vi "Wind_Turbine.vi"() -> (5 "Plug in titles":string[](array[string]), 7 "Plug in values":string[](array[string]))   [LabVIEW 2010]
uses:
  Globals/Meas_global.vi
  Globals/Plug_in_data_global.vi
  Globals/LDA_meas_global_1.vi
  <vilib>/Analysis/NI_AALBase.lvlib
panel:
  in  "Change Dem Voltages?":bool
  out "All WTs":dbl[][](array[numeric]) format="%#.2g"
  out "WT trace index":i32[](array[numeric])
  in  "precision":string
  in  "Add Phase data to results file":bool
  in  "Separation Character":string="\t"
  in  "Output Directory":path
  in  "Save Phase averaged Profiles":bool
  out "LDA Chs":i32[](array[numeric])
  out "WT Stalled?":bool
  out "Pulse No":i32
  out "Last index":i32
  out "subarray":bool[](array[boolean])
  out "Index":i32[](array[numeric])
  out "Pulses per Rev":i32
  out "Av samples per pulse":i32
  out "Threshold":dbl
  in  "Channel to Phase lock":i32[](listbox)
  out "Last Block No of Revs":i32
  out "Hub RPM":dbl
  out "Generator trace":cluster{dbl, dbl, dbl[]}(graph)
  out "Hot wire trace":cluster{dbl, dbl, dbl[][]}(graph)
  out "Number of Revs":i32
  # "Mean RPM      SD RPM           Max-Min"
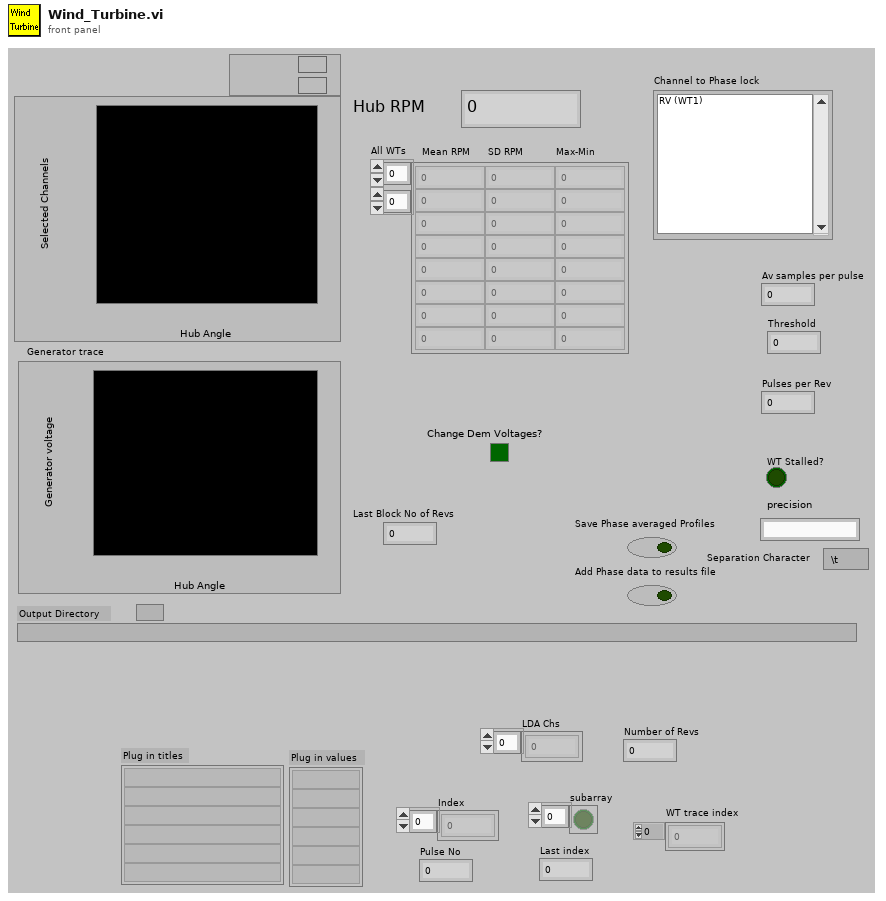
[diagram p1: front panel]
types:
  T1 = typedef "Analysis_info_cluster.ctl" = cluster{"Colour":u32, "Inst type":T2, "Inst name":string, "Symbol":string, "Code name":string, "Extra Info":string, "Inst Array":T3, "Index":i32, "Voltage Index":i32, "Extra Titles":string[], "Extra Values":string[]}
  T2 = typedef "Inst_type.ctl" = enum16{"Propeller anemometer", "Raw voltage", "Pressure Transducer", "Pitot-static tube", "Preston tube", "Hot wire", "Cross wire 1", "Cross wire 2", "Generic Linear", "Generic Polynomial", "Generic BackPoly", "Fast FID", "Thermocouple", "Cold wire", "Pulsed Wire", "LDA Vel", "LDA Tran time", "LDA Arr time"}
  T3 = typedef "Instrument_Array.ctl" = enum16{"PWA", "LDA", "Analogue"}
  T4 = typedef "Post_Process.ctl" = enum16{"Take New Data", "Post Process Raw Data File"}
  T5 = cluster{"[0]":bool, "[1]":bool, "[2]":bool, "[3]":bool}
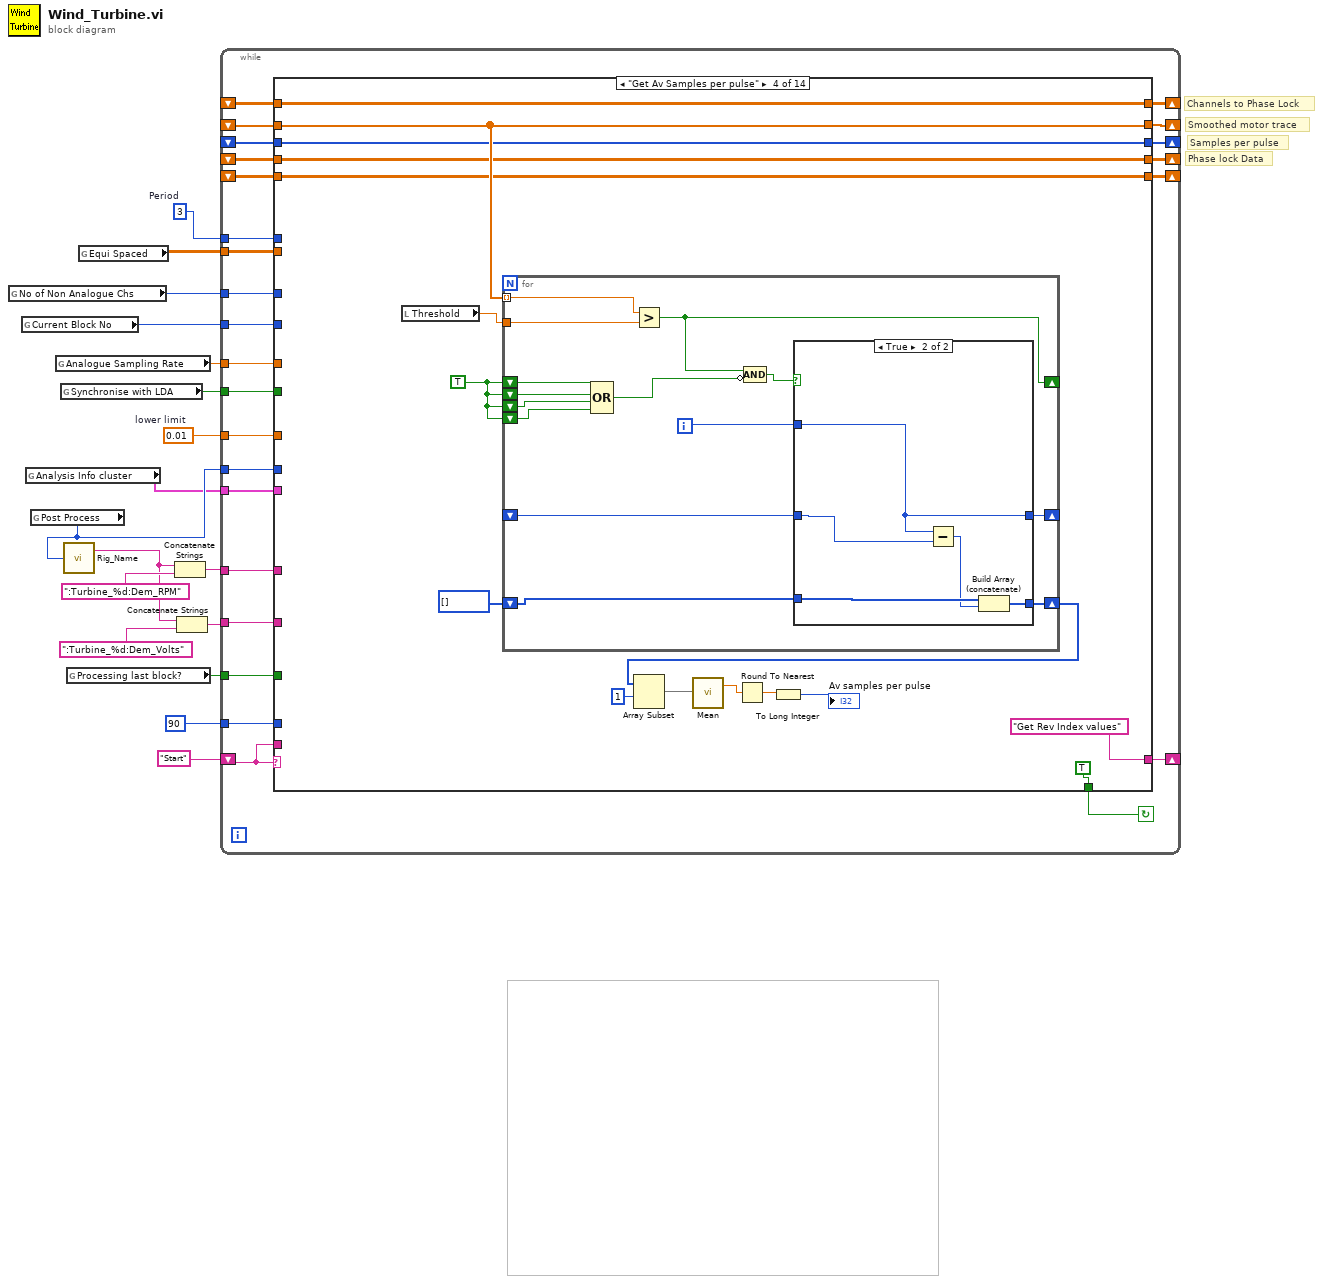
[diagram p0: block diagram]
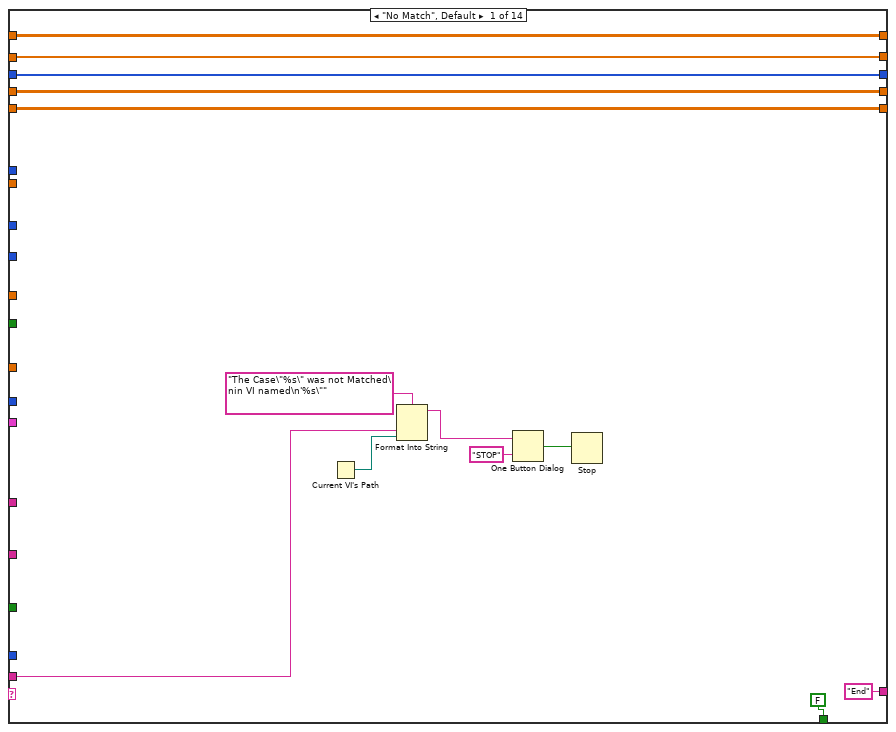
[diagram p2: hidden frame]
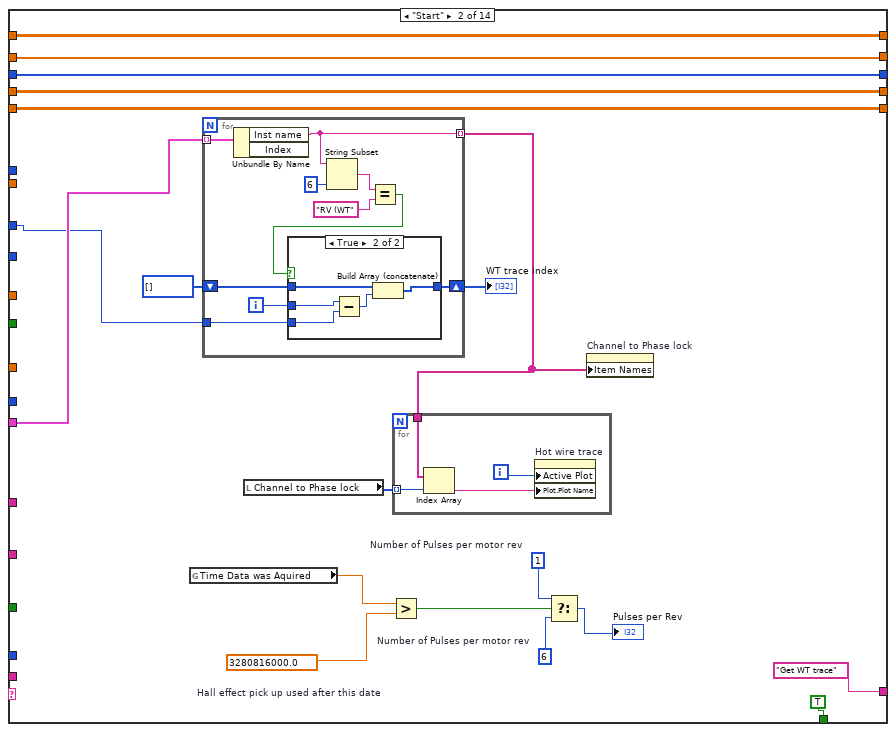
[diagram p3: hidden frame]
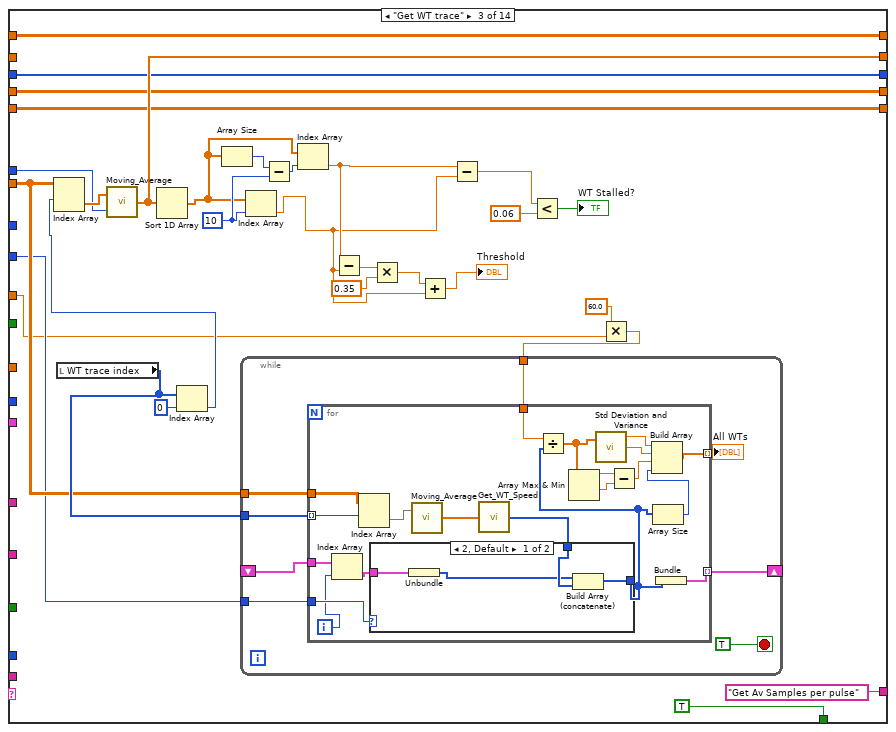
[diagram p5: hidden frame]
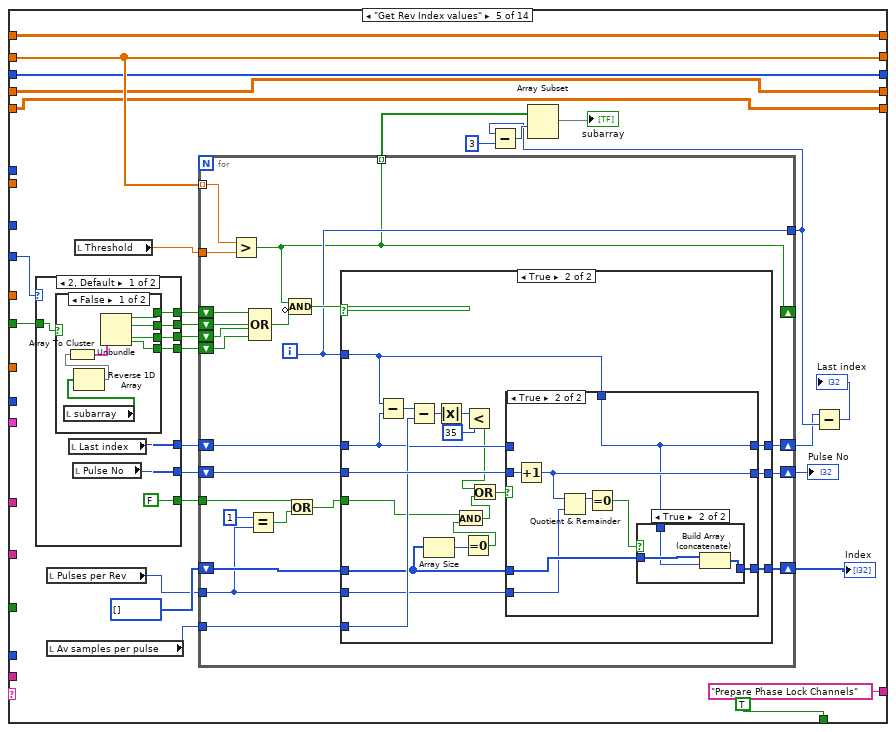
[diagram p8: hidden frame]
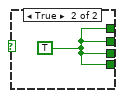
[diagram p9: hidden frame]
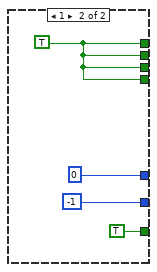
[diagram p10: hidden frame]
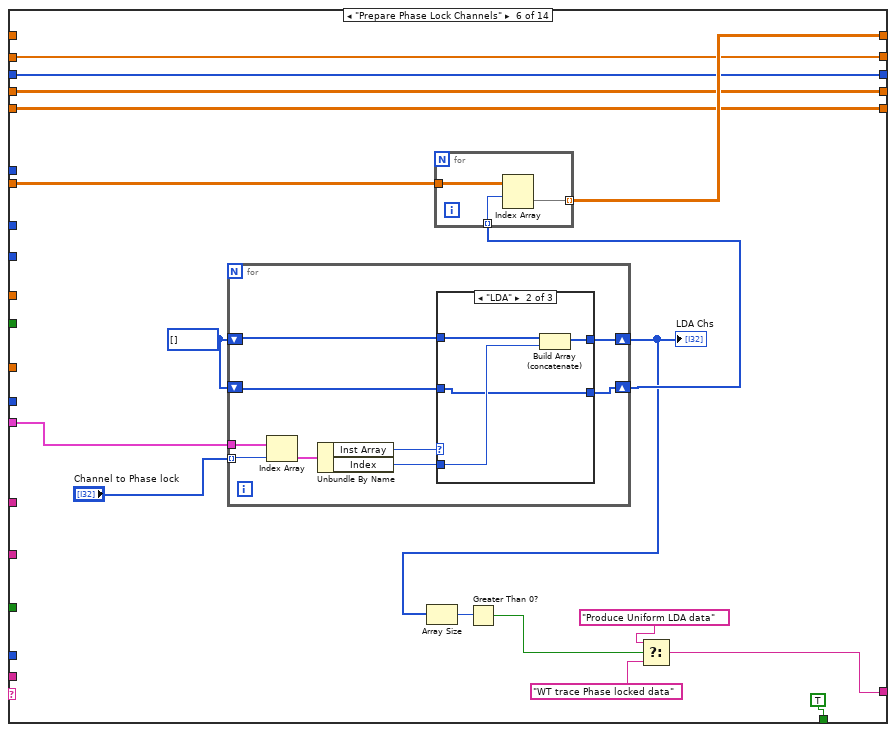
[diagram p14: hidden frame]
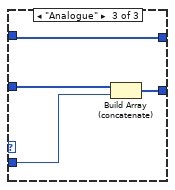
[diagram p16: hidden frame]
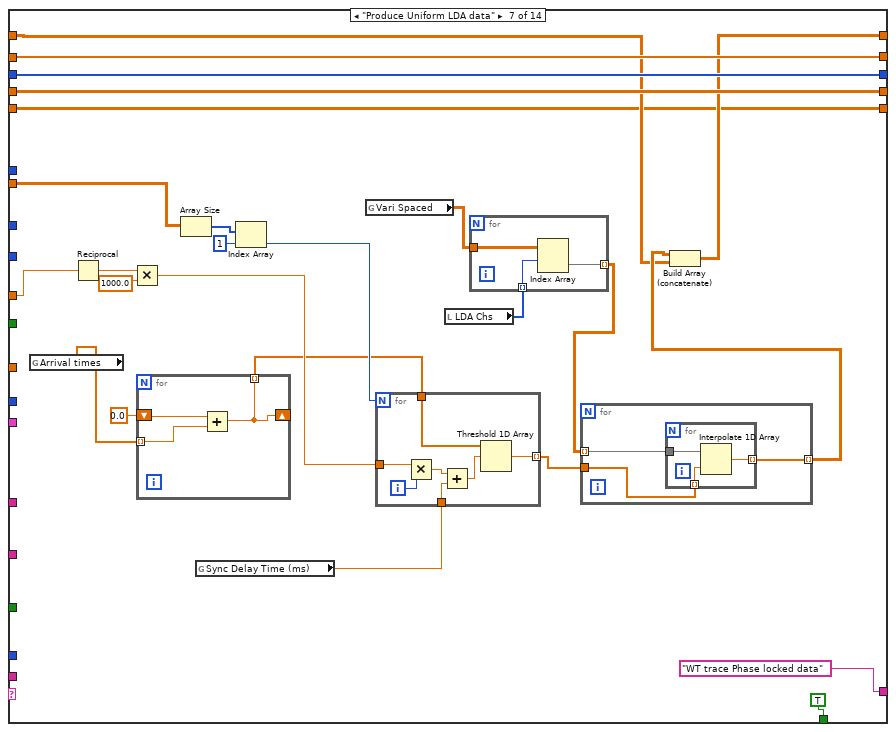
[diagram p17: hidden frame]
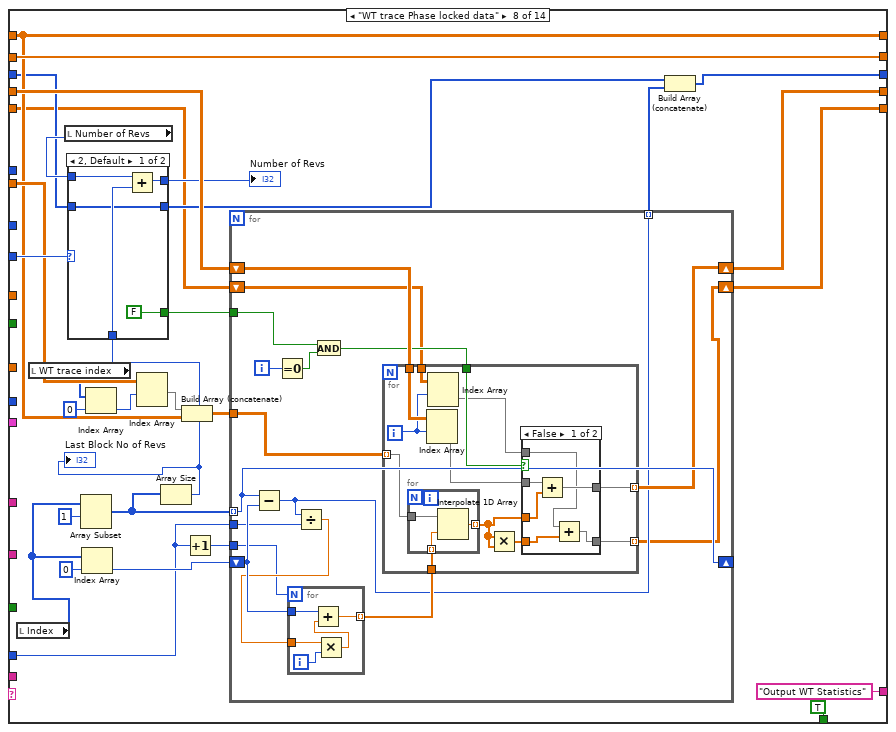
[diagram p18: hidden frame]
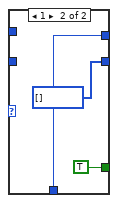
[diagram p19: hidden frame]
diagram:
  w14 = 3  # Period
  w15 = 0.01  # lower limit
  # "Channels to Phase Lock"
  # "Phase lock Data"
  # "Samples per pulse"
  # "Smoothed motor trace"
  n1 = global read "Meas_global.vi" "No of Non Analogue Chs"() -> (w3:i32)
  n2 = global read "Meas_global.vi" "Current Block No"() -> (w17:i32)
  n3 = global read "Meas_global.vi" "Analysis Info cluster"() -> (w6:T1[])
  n4 = global read "Meas_global.vi" "Post Process"() -> (w13:T4)
  n5 = global read "Meas_global.vi" "Analogue Sampling Rate"() -> (w16:dbl)
  n6 = global read "Meas_global.vi" "Synchronise with LDA"() -> (w7:bool)
  n7 = call "Rig_Name.vi"("Post Process"=w13) -> ("Rig Setup before dash"=w9:string)  [unwired: 1 out]
  n8 = global read "Meas_global.vi" "Processing last block?"() -> (w4:bool)
  n9 = global read "Plug_in_data_global.vi" "Equi Spaced"() -> (w2:dbl[][])
  n10 = Concatenate Strings(w9, ":Turbine_%d:Dem_RPM") -> (w8:string)
  n11 = Concatenate Strings(w9, ":Turbine_%d:Dem_Volts") -> (w12:string)
  n12 = while {
    tunnel: w17 -> [w43]
    tunnel: w2 -> [w42]
    shift-right: [w40] -> _
    shift-left: _ -> [w41]
    shift-right: [w39] -> _
    shift-left: _ -> [w38]
    tunnel: w16 -> [w37]
    tunnel: w12 -> [w36]
    tunnel: w8 -> [w35]
    tunnel: w15 -> [w34]
    tunnel: w14 -> [w33]
    tunnel: w13 -> [w32]
    tunnel: w7 -> [w31]
    tunnel: w6 -> [w30]
    shift-right: [w29] -> _
    shift-left: _ -> [w28]
    shift-right: [w27] -> _
    shift-left: "Start" -> [w25]
    tunnel: w4 -> [w24]
    tunnel: w3 -> [w23]
    shift-right: [w22] -> _
    shift-left: _ -> [w21]
    tunnel: 90 -> [w20]
    shift-right: [w18] -> _
    shift-left: _ -> [w19]
    stop <- w26 continue-if-true
    n13 = case shown="\"Get Av Samples per pulse\"" w25 {
      tunnel: w43 -> [_ _ w105 _ w223 _ _ w414 _ _ _ _ _ _]
      tunnel: w42 -> [_ _ w106 _ _ w316 w356 w410 _ _ _ _ _ _]
      tunnel: w41 -> [w48 w64 w112 w161 w200 w312 w365 w409 w485 w529 w570 w597 w671 w685]
      tunnel: [w48 w64 w112 w161 w200 w312 w365 w408 w485 w529 w570 w597 w671 w685] -> w40
      tunnel: [w49 w65 w113 w162 w201 w313 w366 w404 w494 w527 w568 w605 w672 w690] -> w39
      tunnel: w38 -> [w49 w65 w113 w162 w201 w313 w366 w394 w494 w527 w568 w605 w672 w690]
      tunnel: w37 -> [_ _ w103 _ _ _ w359 _ w498 _ _ _ _ w689]
      tunnel: w36 -> [_ _ _ _ _ _ _ _ _ w534 w566 _ _ _]
      tunnel: w35 -> [_ _ _ _ _ _ _ _ _ w533 w541 _ _ _]
      tunnel: w34 -> [_ _ _ _ _ _ _ _ _ _ _ _ _ _]
      tunnel: w33 -> [_ _ w124 _ _ _ _ _ _ _ _ _ _ _]
      tunnel: w32 -> [_ _ _ _ _ _ _ _ _ w532 _ _ _ _]
      tunnel: w31 -> [_ _ _ _ w208 _ _ _ _ _ _ _ _ _]
      tunnel: w30 -> [_ w69 _ _ _ w320 _ _ _ _ _ _ _ _]
      tunnel: [w50 w66 w117 w163 w202 w314 w367 w403 w493 w530 w571 w606 w673 w691] -> w29
      tunnel: w28 -> [w50 w66 _ w163 w202 w314 w367 w403 w493 w530 w571 w606 w673 w691]
      tunnel: ["End" "Get WT trace" "Get Av Samples per pulse" "Get Rev Index values" "Prepare Phase Lock Channels" w308 "WT trace Phase locked data" ("f") "Output WT Statistics" "Get Last Block info" w531 "End" ("f") "Check Folder Name" "Save Phase locked data" "End"] -> w27
      tunnel: [FALSE ("Change Control Voltage?") TRUE ("Processing last block?") TRUE TRUE ("Processing last block?") TRUE ("Change Control Voltage?") TRUE ("Change Control Voltage?") TRUE ("Change Control Voltage?") TRUE ("Change Control Voltage?") TRUE ("Change Control Voltage?") w525 FALSE ("Change Control Voltage?") w602 w663 FALSE ("Change Control Voltage?")] -> w26
      tunnel: w25 -> [w51 _ _ _ _ _ _ _ _ _ _ _ _ _]
      tunnel: w24 -> [_ _ _ _ _ _ _ _ _ w524 _ w600 _ _]
      tunnel: w23 -> [_ w57 _ _ _ _ _ _ _ _ _ _ _ _]
      tunnel: [w45 w63 w111 w160 w197 w315 w345 w398 w486 w528 w569 w604 w670 w688] -> w22
      tunnel: w21 -> [w45 w63 w111 w160 w197 _ w347 w398 w486 w528 w569 w604 w670 w688]
      tunnel: w20 -> [_ _ _ _ _ _ _ w397 w481 _ _ w598 _ w683]
      tunnel: w19 -> [w44 w60 w110 w159 w196 w304 w343 w391 w475 w526 w567 w596 w661 w684]
      tunnel: [w44 w60 w110 w159 w196 w304 w343 w390 w475 w526 w567 w596 w661 w684] -> w18
      frame "No Match", Default {
        n14 = Current VI's Path() -> (path=w52:path)
        n15 = Format Into String(format string="The Case\"%s\" was not Matched\nin VI named\n'%s\"" ("Format String"), w51, w52) -> (resulting string=w55:string)  [unwired: 2 in, 1 out]
        n16 = One Button Dialog(message=w55, button name ("OK")="STOP") -> (true=w53:bool)
        n17 = Stop(stop? (T)=w53) -> ()
      }
      frame "Start" {
        w70 = 6  # Number of Pulses per motor rev
        w71 = 1  # Number of Pulses per motor rev
        w73 = 3280816000.0  # Hall effect pick up used after this date
        n18 = global read "Meas_global.vi" "Time Data was Aquired"() -> (w74:dbl)
        n19 = for {
          tunnel: w69 -> [w89] mode=indexing
          tunnel: [w88] -> w62 mode=indexing
          shift-right: [w82] -> w58
          shift-left: i32[] [] -> [w83]
          tunnel: w57 -> [w80]
          i -> [w81]
          n20 = Unbundle By Name(w89) -> ("Inst name"=w88:string)  [unwired: 1 out]
          n21 = String Subset(string=w88, length (rest)=6 ("length (rest)")) -> (substring=w85:string)  [unwired: 1 out]
          n22 = Equal?(x=w85, y="RV (WT") -> (x = y?=w84:bool)
          n23 = case shown="True" w84 {
            tunnel: w83 -> [w90 w95]
            tunnel: [w90 w94] -> w82
            tunnel: w81 -> [_ w93]
            tunnel: w80 -> [_ w91]
            frame False {
            }
            frame True {
              n24 = Subtract(x=w93, y=w91) -> (x-y=w92:i32)
              n25 = Build Array (concatenate)(w95, w92) -> (w94:i32[])
            }
          }
        }
        "WT trace index" <- w58
        n26 = local read "Channel to Phase lock"() -> (w61:i32[])
        n27 = Greater?(x=w74, y=w73) -> (0:w72:bool)
        n28 = for {
          tunnel: w62 -> [w79]
          tunnel: w61 -> [w78] mode=indexing
          i -> [w77]
          n29 = Index Array(array=w79, index=w78) -> (element=w76:string)
          n30 = property on="Hot wire trace" class="WFGraph (strict)"("Active Plot"=w77, "Plot.Plot Name"=w76) -> ()  [unwired: 2 in, 2 out]
        }
        n31 = Select(t=w71, s=w72, f=w70) -> (s? t:f=→"Pulses per Rev":i32)
        n32 = property on="Channel to Phase lock" class="LstBox (strict)"("Item Names"=w62) -> ()  [unwired: 2 in, 2 out]
      }
      frame "Get WT trace" {
        w122 = 10 ("index")
        n33 = local read "WT trace index"() -> (w107:i32[])
        n34 = Index Array(array=w107, index=0) -> (element=w108:i32)
        n35 = Index Array(array=w106, index (row)=w108) -> (element=w125:dbl[])  [unwired: 1 in]
        n36 = call "Moving_Average.vi"("Period"=w124, "Input Array"=w125) -> ("N+1-Period"=w117:dbl[])
        n37 = Sort 1D Array(array=w117) -> (sorted array=w120:dbl[])
        n38 = Array Size(array=w120) -> (size(s)=w123:i32)
        n39 = Index Array(array=w120, index=w122) -> (element=w97:dbl)
        n40 = Subtract(x=w123, y=w122) -> (x-y=w121:i32)
        n41 = Index Array(array=w120, index=w121) -> (element=w98:dbl)
        n42 = Subtract(x=w98, y=w97) -> (x-y=w101:dbl)
        n43 = Multiply(x=w101, y=0.35) -> (x*y=w99:dbl)
        n44 = Add(x=w99, y=w97) -> (x+y=→"Threshold":dbl)
        n45 = Subtract(x=w98, y=w97) -> (x-y=w118:dbl)
        n46 = Less?(x=w118, y=0.06) -> (x < y?=→"WT Stalled?":bool)
        n47 = Multiply(x=60.0, y=w103) -> (x*y=w102:dbl)
        n48 = while {
          tunnel: w107 -> [w133]
          tunnel: w106 -> [w132]
          tunnel: w105 -> [w131]
          shift-right: [w126] -> _
          shift-left: _ -> [w130]
          tunnel: w102 -> [w129]
          stop <- TRUE stop-if-true
          n49 = for {
            tunnel: w133 -> [w152] mode=indexing
            tunnel: w132 -> [w151]
            tunnel: w131 -> [w149]
            tunnel: w130 -> [w139]
            tunnel: w129 -> [w147]
            tunnel: [w140] -> w127 mode=indexing
            tunnel: [w134] -> w126 mode=indexing
            i -> [w138]
            n50 = Index Array(array=w139, index=w138) -> (element=w137:cluster{"Samples per pulse":i32[]})
            n51 = Index Array(array=w151, index (row)=w152) -> (element=w153:dbl[])  [unwired: 1 in]
            n52 = call "Moving_Average.vi"("Input Array"=w153) -> ("N+1-Period"=w150:dbl[])  [unwired: 1 in]
            n53 = call "Get_WT_Speed.vi"("Opto Trace"=w150) -> ("Samples per pulse"=w148:i32[])
            n54 = case shown="2, Default" w149 {
              tunnel: [w156 w158] -> w135
              tunnel: w148 -> [w157 w158]
              tunnel: w137 -> [w155 _]
              frame 2, Default {
                n55 = Unbundle(w155) -> ("Samples per pulse"=w154:i32[])
                n56 = Build Array (concatenate)(w154, w157) -> (w156:i32[])
              }
              frame 1 {
              }
            }
            n57 = Divide(x=w147, y=w135) -> (x/y=w144:dbl[])
            n58 = Array Max & Min(array=w144) -> (max value=w146:dbl, min value=w145:dbl)  [unwired: 2 out]
            n59 = call <vilib>:"Std Deviation and Variance.vi"("X"=w144) -> ("mean"=w143:dbl, "standard deviation"=w142:dbl)  [unwired: 1 in, 1 out]
            n60 = Subtract(x=w146, y=w145) -> (x-y=w141:dbl)
            n61 = Array Size(array=w135) -> (size(s)=w136:i32)
            n62 = Build Array(w143, w142, w141, w136) -> (w140:dbl[])
            n63 = Bundle("Samples per pulse"=w135) -> (w134:cluster{"Samples per pulse":i32[]})  [unwired: 1 in]
          }
          "All WTs" <- w127
        }
      }
      frame "Get Av Samples per pulse" {
        w172 = TRUE
        n64 = local read "Threshold"() -> (w166:dbl)
        n65 = for {
          shift-right: [w175] -> _
          shift-left: w172 -> [w180]
          shift-right: [w185] -> _
          shift-left: _ -> [w184]
          tunnel: w163 -> [w188] mode=indexing
          tunnel: w166 -> [w187]
          shift-right: [w182] -> w171
          shift-left: i32[] [] -> [w183]
          shift-left: w172 -> [w179]
          shift-left: w172 -> [w178]
          shift-left: w172 -> [w176]
          i -> [w181]
          n66 = Compound Arithmetic op=OR(w180, w179, w178, w176) -> (w177:bool)
          n67 = Greater?(x=w188, y=w187) -> (0:w175:bool)
          n68 = Compound Arithmetic op=AND(w175, invert w177) -> (w186:bool)
          n69 = case shown="True" w186 {
            tunnel: [w190 w193] -> w185
            tunnel: w181 -> [_ w193]
            tunnel: w184 -> [w190 w192]
            tunnel: w183 -> [w189 w195]
            tunnel: [w189 w194] -> w182
            frame False {
            }
            frame True {
              n70 = Subtract(x=w193, y=w192) -> (x-y=w191:i32)
              n71 = Build Array (concatenate)(w195, w191) -> (w194:i32[])
            }
          }
        }
        n72 = Array Subset(array=w171, index=1) -> (w169:i32[])  [unwired: 1 in]
        n73 = call <vilib>:"Mean.vi"("X"=w169) -> ("mean"=w168:dbl)  [unwired: 1 out]
        n74 = Round To Nearest(number=w168) -> (nearest integer value=w167:dbl)
        n75 = To Long Integer(number=w167) -> (32bit integer=→"Av samples per pulse":i32)
      }
      frame "Get Rev Index values" {
        n76 = case shown="2, Default" w223 {
          tunnel: [w225 -1] -> w222
          tunnel: [w226 0] -> w220
          tunnel: [w232 w241] -> w215
          tunnel: [w231 w241] -> w214
          tunnel: [w230 w241] -> w213
          tunnel: [w229 w241] -> w212
          tunnel: [FALSE TRUE] -> w211
          tunnel: w208 -> [w227 _]
          frame 2, Default {
            n77 = case shown="False" w227 {
              tunnel: [w237 w240] -> w232
              tunnel: [w236 w240] -> w231
              tunnel: [w235 w240] -> w230
              tunnel: [w234 w240] -> w229
              frame False {
                n78 = local read "subarray"() -> (w233:bool[])
                n79 = Reverse 1D Array(array=w233) -> (reversed array=w239:bool[])
                n80 = Array To Cluster(array=w239) -> (cluster=w238:T5)
                n81 = Unbundle(w238) -> ("[0]"=w237:bool, "[1]"=w236:bool, "[2]"=w235:bool, "[3]"=w234:bool)
              }
              frame True {
                w240 = TRUE ("[0]")
              }
            }
            n82 = local read "Last index"() -> (w226:i32)
            n83 = local read "Pulse No"() -> (w225:i32)
          }
          frame 1 {
            w241 = TRUE
          }
        }
        n84 = local read "Pulses per Rev"() -> (w205:i32)
        n85 = local read "Av samples per pulse"() -> (w206:i32)
        n86 = local read "Threshold"() -> (w207:dbl)
        n87 = for {
          shift-right: [w252] -> _
          shift-left: w215 -> [w256]
          shift-right: [w263] -> w209
          shift-left: w220 -> [w260]
          tunnel: w202 -> [w266] mode=indexing
          tunnel: w207 -> [w265]
          shift-right: [w261] -> w203
          shift-left: w222 -> [w262]
          shift-right: [w258] -> w204
          shift-left: i32[] [] -> [w259]
          tunnel: [w257] -> w210
          shift-left: w214 -> [w255]
          shift-left: w213 -> [w254]
          tunnel: [w252] -> w217 mode=indexing
          shift-left: w212 -> [w251]
          tunnel: w206 -> [w250]
          tunnel: w211 -> [w246]
          tunnel: w205 -> [w249]
          i -> [w257]
          n88 = Greater?(x=w266, y=w265) -> (0:w252:bool)
          n89 = Equal?(x=1, y=w249) -> (x = y?=w247:bool)
          n90 = Compound Arithmetic op=OR(w256, w255, w254, w251) -> (w253:bool)
          n91 = Or(x=w246, y=w247) -> (x .or. y?=w245:bool)
          n92 = Compound Arithmetic op=AND(w252, invert w253) -> (w264:bool)
          n93 = case shown="True" w264 {
            tunnel: [w269 w279] -> w263
            tunnel: w257 -> [_ w285]
            tunnel: w262 -> [w268 w288]
            tunnel: [w268 w287] -> w261
            tunnel: w260 -> [w269 w278]
            tunnel: w259 -> [w267 w277]
            tunnel: [w267 w286] -> w258
            tunnel: w250 -> [_ w283]
            tunnel: w245 -> [_ w272]
            tunnel: w249 -> [_ w271]
            frame False {
            }
            frame True {
              n94 = Subtract(x=w285, y=w278) -> (x-y=w284:i32)
              n95 = Subtract(x=w284, y=w283) -> (x-y=w282:i32)
              n96 = Array Size(array=w277) -> (size(s)=w275:i32)
              n97 = Absolute Value(x=w282) -> (abs(x)=w281:i32)
              n98 = Equal To 0?(x=w275) -> (x = 0?=w274:bool)
              n99 = And(x=w272, y=w274) -> (x .and. y?=w273:bool)
              n100 = Less?(x=w281, y=35) -> (x < y?=w270:bool)
              n101 = Or(x=w270, y=w273) -> (x .or. y?=w276:bool)
              n102 = case shown="True" w276 {
                tunnel: w288 -> [w291 w299]
                tunnel: [w291 w298] -> w287
                tunnel: w277 -> [w290 w295]
                tunnel: [w290 w294] -> w286
                tunnel: w285 -> [_ w293]
                tunnel: [w289 w293] -> w279
                tunnel: w278 -> [w289 _]
                tunnel: w271 -> [_ w292]
                frame False {
                }
                frame True {
                  n103 = Increment(x=w299) -> (x+1=w298:i32)
                  n104 = Quotient & Remainder(x=w298, y=w292) -> (x-y*floor(x/y)=w297:i32)  [unwired: 1 out]
                  n105 = Equal To 0?(x=w297) -> (x = 0?=w296:bool)
                  n106 = case shown="True" w296 {
                    tunnel: w295 -> [w300 w303]
                    tunnel: w293 -> [_ w302]
                    tunnel: [w300 w301] -> w294
                    frame False {
                    }
                    frame True {
                      n107 = Build Array (concatenate)(w303, w302) -> (w301:i32[])
                    }
                  }
                }
              }
            }
          }
        }
        "Index" <- w204
        "Pulse No" <- w203
        n108 = Subtract(x=w210, y=3) -> (x-y=w218:i32)
        n109 = Array Subset(array=w217, index=w218) -> (→"subarray":bool[])  [unwired: 1 in]
        n110 = Subtract(x=w209, y=w210) -> (x-y=→"Last index":i32)
      }
      frame "Prepare Phase Lock Channels" {
        w318 = i32[] []
        n111 = for {
          tunnel: "Channel to Phase lock" -> [w332] mode=indexing
          tunnel: w320 -> [w331]
          shift-right: [w324] -> w317
          shift-left: w318 -> [w325]
          shift-right: [w326] -> w310
          shift-left: w318 -> [w327]
          n112 = Index Array(array=w331, index=w332) -> (element=w330:T1)
          n113 = Unbundle By Name(w330) -> ("Inst Array"=w329:T3, "Index"=w328:i32)
          n114 = case shown="\"LDA\"" w329 {
            tunnel: w328 -> [_ w338 w342]
            tunnel: w327 -> [w334 w337 w339]
            tunnel: [w334 w336 w339] -> w326
            tunnel: w325 -> [w333 w335 w341]
            tunnel: [w333 w335 w340] -> w324
            frame "PWA" {
            }
            frame "LDA" {
              n115 = Build Array (concatenate)(w337, w338) -> (w336:i32[])
            }
            frame "Analogue" {
              n116 = Build Array (concatenate)(w341, w342) -> (w340:i32[])
            }
          }
        }
        "LDA Chs" <- w310
        n117 = Array Size(array=w310) -> (size(s)=w311:i32)
        n118 = for {
          tunnel: w317 -> [w323] mode=indexing
          tunnel: w316 -> [w322]
          tunnel: [w321] -> w315 mode=indexing
          n119 = Index Array(array=w322, index (row)=w323) -> (element=w321:dbl[])  [unwired: 1 in]
        }
        n120 = Greater Than 0?(x=w311) -> (x > 0?=w309:bool)
        n121 = Select(t="Produce Uniform LDA data", s=w309, f="WT trace Phase locked data") -> (s? t:f=w308:string)
      }
      frame "Produce Uniform LDA data" {
        n122 = global read "LDA_meas_global_1.vi" "Arrival times"() -> (w361:dbl[])
        n123 = Reciprocal(x=w359) -> (1/x=w360:dbl)
        n124 = Multiply(x=w360, y=1000.0) -> (x*y=w357:dbl)
        n125 = for {
          shift-right: [w381] -> _
          shift-left: 0.0 -> [w383]
          tunnel: w361 -> [w382] mode=indexing
          tunnel: [w381] -> w346 mode=indexing
          n126 = Add(x=w383, y=w382) -> (x+y=w381:dbl)
        }
        n127 = Array Size(array=w356) -> (size(s)=w355:i32[])
        n128 = global read "LDA_meas_global_1.vi" "Sync Delay Time (ms)"() -> (w344:dbl)
        n129 = Index Array(array=w355, index=1) -> (element=w353:i32)
        n130 = global read "Plug_in_data_global.vi" "Vari Spaced"() -> (w350:dbl[][])
        n131 = for {
          N: w353 -> [_]
          tunnel: w357 -> [w379]
          tunnel: w346 -> [w378]
          tunnel: [w377] -> w352 mode=indexing
          tunnel: w344 -> [w374]
          i -> [w380]
          n132 = Multiply(x=w379, y=w380) -> (x*y=w376:dbl)
          n133 = Add(x=w376, y=w374) -> (x+y=w375:dbl)
          n134 = Threshold 1D Array(2:w375, 3:w378) -> (0:w377:dbl)  [unwired: 1 out]
        }
        n135 = local read "LDA Chs"() -> (w351:i32[])
        n136 = for {
          tunnel: w351 -> [w386] mode=indexing
          tunnel: w350 -> [w385]
          tunnel: [w384] -> w349 mode=indexing
          n137 = Index Array(array=w385, index (row)=w386) -> (element=w384:dbl[])  [unwired: 1 in]
        }
        n138 = for {
          tunnel: [w370] -> w348 mode=indexing
          tunnel: w349 -> [w369] mode=indexing
          tunnel: w352 -> [w368]
          n139 = for {
            tunnel: [w373] -> w370 mode=indexing
            tunnel: w369 -> [w372]
            tunnel: w368 -> [w371] mode=indexing
            n140 = Interpolate 1D Array(1:w371, 2:w372) -> (0:w373:dbl)
          }
        }
        n141 = Build Array (concatenate)(w348, w347) -> (w345:dbl[][])
      }
      frame "WT trace Phase locked data" {
        n142 = local read "Index"() -> (w406:i32[])
        n143 = local read "WT trace index"() -> (w389:i32[])
        n144 = local read "Number of Revs"() -> (w407:i32)
        n145 = Array Subset(array=w406, index=1) -> (w413:i32[])  [unwired: 1 in]
        n146 = Index Array(array=w406, index=0) -> (element=w412:i32)
        n147 = Index Array(array=w389, index=0) -> (element=w387:i32)
        n148 = Index Array(array=w410, index (row)=w387) -> (element=w400:dbl[])  [unwired: 1 in]
        n149 = Array Size(array=w413) -> (size(s)=w392:i32)
        "Last Block No of Revs" <- w392
        n150 = case shown="2, Default" w414 {
          tunnel: [w419 w424] -> w405
          tunnel: w392 -> [w420 w424]
          tunnel: w407 -> [w421 _]
          tunnel: [FALSE TRUE] -> w411
          tunnel: [w417 i32[] []] -> w395
          tunnel: w394 -> [w417 _]
          frame 2, Default {
            n151 = Add(x=w421, y=w420) -> (x+y=w419:i32)
          }
          frame 1 {
          }
        }
        "Number of Revs" <- w405
        n152 = Build Array (concatenate)(w400, w398) -> (w399:dbl[][])
        n153 = Increment(x=w397) -> (x+1=w396:i32)
        n154 = for {
          shift-right: [w440] -> _
          shift-left: w412 -> [w433]
          tunnel: w413 -> [w440] mode=indexing
          tunnel: w411 -> [w437]
          shift-right: [w435] -> w408
          shift-left: w409 -> [w434]
          tunnel: w399 -> [w436]
          tunnel: w396 -> [w431]
          tunnel: w397 -> [w430]
          tunnel: [w427] -> w393 mode=indexing
          shift-right: [w425] -> w390
          shift-left: w391 -> [w426]
          i -> [w439]
          n155 = Subtract(x=w440, y=w433) -> (x-y=w427:i32)
          n156 = Equal To 0?(x=w439) -> (x = 0?=w438:bool)
          n157 = Divide(x=w427, y=w430) -> (x/y=w432:dbl)
          n158 = for {
            N: w431 -> [_]
            tunnel: w433 -> [w445]
            tunnel: w432 -> [w443]
            tunnel: [w441] -> w429 mode=indexing
            i -> [w444]
            n159 = Multiply(x=w443, y=w444) -> (x*y=w442:dbl)
            n160 = Add(x=w445, y=w442) -> (x+y=w441:dbl)
          }
          n161 = And(x=w437, y=w438) -> (x .and. y?=w428:bool)
          n162 = for {
            tunnel: w436 -> [w454] mode=indexing
            tunnel: w428 -> [w457]
            tunnel: [w456] -> w435 mode=indexing
            tunnel: w434 -> [w452]
            tunnel: w429 -> [w453]
            tunnel: w426 -> [w451]
            tunnel: [w448] -> w425 mode=indexing
            i -> [w450]
            n163 = for {
              tunnel: w454 -> [w460]
              tunnel: [w459] -> w449 mode=indexing
              tunnel: w453 -> [w458] mode=indexing
              n164 = Interpolate 1D Array(1:w458, 2:w460) -> (0:w459:dbl)
            }
            n165 = Index Array(array=w452, index (row)=w450) -> (element=w455:dbl[])  [unwired: 1 in]
            n166 = Index Array(array=w451, index (row)=w450) -> (element=w446:dbl[])  [unwired: 1 in]
            n167 = Multiply(x=w449, y=w449) -> (x*y=w447:dbl[])
            n168 = case shown="False" w457 {
              tunnel: [w466 w468] -> w456
              tunnel: w449 -> [w464 w468]
              tunnel: w455 -> [w465 _]
              tunnel: [w462 w467] -> w448
              tunnel: w447 -> [w463 w467]
              tunnel: w446 -> [w461 _]
              frame False {
                n169 = Add(x=w465, y=w464) -> (x+y=w466:dbl[])
                n170 = Add(x=w461, y=w463) -> (x+y=w462:dbl[])
              }
              frame True {
              }
            }
          }
        }
        n171 = Build Array (concatenate)(w395, w393) -> (w404:i32[])
      }
      frame "Output WT Statistics" {
        w471 = string[] []
        n172 = Multiply(x=60.0, y=w498) -> (x*y=w497:dbl)
        n173 = Divide(x=360, y=w481) -> (x/y=w476:dbl)
        n174 = Divide(x=w497, y=w494) -> (x/y=w496:dbl[])
        n175 = call <vilib>:"Std Deviation and Variance.vi"("X"=w496) -> ("mean"=→"Hub RPM":dbl)  [unwired: 1 in, 2 out]
        n176 = local read "All WTs"() -> (w473:dbl[][])
        n177 = for {
          tunnel: w473 -> [w511] mode=indexing
          shift-right: [w505] -> w472
          shift-left: w471 -> [w506]
          shift-right: [w501] -> w469
          shift-left: w471 -> [w503]
          tunnel: string[] ["WT_%d:Hub_RPM:Mean", "WT_%d:Hub_RPM:St_Dev", "WT_%d:Hub_RPM:Max-Min", "WT_%d:Number_of:Revs"] ("Plug in titles") -> [w504]
          i -> [w500]
          n178 = Index Array(array=w511, index=0) -> (element=w510:dbl)
          n179 = Index Array(array=w511, index=1) -> (element=w509:dbl)
          n180 = Index Array(array=w511, index=2) -> (element=w508:dbl)
          n181 = Index Array(array=w511, index=3) -> (element=w507:dbl)
          n182 = for {
            tunnel: w504 -> [w523] mode=indexing
            tunnel: [w521] -> w502 mode=indexing
            tunnel: w500 -> [w520]
            n183 = Increment(x=w520) -> (x+1=w522:i32)
            n184 = Format Into String(format string=w523, w522) -> (resulting string=w521:string)  [unwired: 2 in, 1 out]
          }
          n185 = call "Number_2_string.vi"("number"=w510) -> ("String"=w518:string)  [unwired: 1 in]
          n186 = call "Number_2_string.vi"("number"=w509) -> ("String"=w519:string)  [unwired: 1 in]
          n187 = call "Number_2_string.vi"("number"=w508) -> ("String"=w517:string)  [unwired: 1 in]
          n188 = Number To Decimal String(number=w507) -> (decimal integer string=w516:string)  [unwired: 1 out]
          n189 = Build Array (concatenate)(w506, w518, w519, w517, w516) -> (w505:string[])
          n190 = Build Array (concatenate)(w503, w502) -> (w501:string[])
        }
        "Plug in titles" <- w469
        "Plug in values" <- w472
        n191 = local read "Number of Revs"() -> (w474:i32)
        n192 = Index Array(array=w485, index (row)=0 ("index")) -> (element=w489:dbl[])  [unwired: 1 in]
        n193 = Array Subset(array=w485, index (row)=1 ("index")) -> (w487:dbl[][])  [unwired: 3 in]
        n194 = Divide(x=w487, y=w474) -> (x/y=w484:dbl[][])
        n195 = Divide(x=w489, y=w474) -> (x/y=w478:dbl[])
        n196 = Bundle(0.0, w476, w484) -> (→"Hot wire trace":cluster{dbl, dbl, dbl[][]})  [unwired: 1 out]
        n197 = Bundle(0.0, w476, w478) -> (→"Generator trace":cluster{dbl, dbl, dbl[]})  [unwired: 1 out]
      }
      frame "Get Last Block info" {
        n198 = case shown="\"Take New Data\"" w532 {
          tunnel: w534 -> [_ _]
          tunnel: w533 -> [_ _]
          tunnel: ["Change Dem Volts" "Post Process"] -> w531
          tunnel: [w537 TRUE ("Processing last block?")] -> w525
          tunnel: w524 -> [w535 _]
          frame "Take New Data" {
            n199 = And(x="Change Dem Voltages?", y=w535) -> (x .and. y?=w537:bool)
          }
          frame "Post Process Raw Data File" {
          }
        }
      }
      frame "Change Dem Volts" {
        n200 = local read "All WTs"() -> (w562:dbl[][])
        n201 = for {
          tunnel: w566 -> [w594]
          tunnel: [w593] -> w565 mode=indexing
          tunnel: [w592] -> w548 mode=indexing
          tunnel: w562 -> [w590] mode=indexing
          tunnel: [w589] -> w560 mode=indexing
          tunnel: [w588] -> w542
          tunnel: w541 -> [w587]
          i -> [w595]
          n202 = Increment(x=w595) -> (x+1=w588:i32)
          n203 = Format Into String(format string=w594, w588) -> (resulting string=w592:string)  [unwired: 2 in, 1 out]
          n204 = Format Into String(format string=w587, w588) -> (resulting string=w593:string)  [unwired: 2 in, 1 out]
          n205 = Index Array(array=w590, index=0) -> (element=w589:dbl)
        }
        n206 = Build Array (concatenate)(w565, w548) -> (w564:string[])
        n207 = call "Get_Current_Scan_client.vi"("ADAM Ch Names"=w564) -> ("Numerical Values"=w563:dbl[])  [unwired: 3 out]
        n208 = Split 1D Array(array=w563, index=w542) -> (first subarray=w561:dbl[], second subarray=w559:dbl[])
        n209 = Divide(x=w561, y=w560) -> (x/y=w551:dbl[])
        n210 = In Range and Coerce(upper limit=1.05, x=w551, lower limit=0.95) -> (coerced(x)=w550:dbl[], In Range?=w549:bool[])
        n211 = Multiply(x=w550, y=w559) -> (x*y=w554:dbl[])
        n212 = In Range and Coerce(upper limit=9.9, x=w554, lower limit=0.0) -> (coerced(x)=w547:dbl[])  [unwired: 1 out]
        n213 = for {
          shift-right: [w576] -> w545
          shift-left: string[] [] -> [w577]
          shift-right: [w574] -> w546
          shift-left: dbl[] [] -> [w575]
          tunnel: w549 -> [w578] mode=indexing
          tunnel: w548 -> [w573] mode=indexing
          tunnel: w547 -> [w572] mode=indexing
          n214 = case shown="False" w578 {
            tunnel: w577 -> [w580 w586]
            tunnel: [w580 w585] -> w576
            tunnel: w575 -> [w579 w584]
            tunnel: [w579 w583] -> w574
            tunnel: w573 -> [_ w582]
            tunnel: w572 -> [_ w581]
            frame False {
            }
            frame True {
              n215 = Build Array (concatenate)(w586, w582) -> (w585:string[])
              n216 = Build Array (concatenate)(w584, w581) -> (w583:dbl[])
            }
          }
        }
        n217 = call "ASYNC_Adam_client.vi"("Values"=w546, "Channel Names"=w545) -> ()  [unwired: 2 out]
      }
      frame "Post Process" {
        n218 = Compound Arithmetic op=AND("Add Phase data to results file", w600) -> (w599:bool)
        n219 = case shown="True" w599 {
          tunnel: w598 -> [_ w610]
          tunnel: w597 -> [_ w609]
          tunnel: w596 -> [_ w608]
          frame False {
          }
          frame True {
            n220 = stacked-sequence {
              tunnel: w610 -> [w612 _]
              tunnel: w609 -> [_ w639]
              tunnel: w608 -> [_ w643]
              frame #0 {
                n221 = local read "Channel to Phase lock"() -> (w619:i32[])
                n222 = property on="Channel to Phase lock" class="LstBox (strict)"() -> ("Item Names"=w618:string[])  [unwired: 2 in, 2 out]
                n223 = local read "Plug in titles"() -> (w613:string[])
                n224 = Divide(x=360, y=w612) -> (x/y=w615:dbl)
                n225 = Increment(x=w612) -> (x+1=w611:i32)
                n226 = for {
                  tunnel: w618 -> [w637]
                  tunnel: w619 -> [w636] mode=indexing
                  tunnel: [w635] -> w617 mode=indexing
                  n227 = Index Array(array=w637, index=w636) -> (element=w635:string)
                }
                n228 = for {
                  tunnel: w617 -> [w626] mode=indexing
                  tunnel: w615 -> [w625]
                  shift-right: [w622] -> w614
                  shift-left: w613 -> [w624]
                  tunnel: w611 -> [w620]
                  n229 = for {
                    N: w620 -> [_]
                    tunnel: w626 -> [w628]
                    tunnel: w625 -> [w633]
                    tunnel: [w631] -> w623 mode=indexing
                    tunnel: [w627] -> w621 mode=indexing
                    i -> [w634]
                    n230 = Multiply(x=w633, y=w634) -> (x*y=w629:dbl)
                    n231 = Format Into String(format string="%s:Mean:%.1f Deg", w628, w629) -> (resulting string=w631:string)  [unwired: 2 in, 1 out]
                    n232 = Format Into String(format string="%s:Variance:%.1f Deg", w628, w629) -> (resulting string=w627:string)  [unwired: 2 in, 1 out]
                  }
                  n233 = Build Array (concatenate)(w624, w623, w621) -> (w622:string[])
                }
                n234 = local write "Plug in titles"(w614) -> ()
              }
              frame #1 {
                n235 = local read "Number of Revs"() -> (w646:i32)
                n236 = Array Subset(array=w643, index (row)=1 ("index")) -> (w641:dbl[][])  [unwired: 3 in]
                n237 = Array Subset(array=w639, index (row)=1 ("index")) -> (w638:dbl[][])  [unwired: 3 in]
                n238 = local read "Plug in values"() -> (w648:string[])
                n239 = Divide(x=w638, y=w646) -> (x/y=w647:dbl[][])
                n240 = Divide(x=w641, y=w646) -> (x/y=w644:dbl[][])
                n241 = for {
                  tunnel: w647 -> [w654] mode=indexing
                  shift-right: [w652] -> w645
                  shift-left: w648 -> [w653]
                  tunnel: w644 -> [w650] mode=indexing
                  n242 = for {
                    tunnel: w654 -> [w659] mode=indexing
                    tunnel: [w660] -> w651 mode=indexing
                    tunnel: w650 -> [w658] mode=indexing
                    tunnel: [w655] -> w649 mode=indexing
                    n243 = Multiply(x=w659, y=w659) -> (x*y=w657:dbl)
                    n244 = Subtract(x=w658, y=w657) -> (x-y=w656:dbl)
                    n245 = call "Number_2_string.vi"("number"=w659) -> ("String"=w660:string)  [unwired: 1 in]
                    n246 = call "Number_2_string.vi"("number"=w656) -> ("String"=w655:string)  [unwired: 1 in]
                  }
                  n247 = Build Array (concatenate)(w653, w651, w649) -> (w652:string[])
                }
                n248 = local write "Plug in values"(w645) -> ()
              }
            }
          }
        }
        n249 = Compound Arithmetic op=AND("Save Phase averaged Profiles", w600) -> (w602:bool)
      }
      frame "Check Folder Name" {
        n250 = File/Directory Info(path="Output Directory") -> (error out=w666:errorcluster)  [unwired: 1 in, 6 out]
        n251 = Empty String/Path?(string/path="Output Directory") -> (empty?=w668:bool)
        n252 = Unbundle By Name(w666) -> ("status"=w667:bool)
        n253 = Or(x=w668, y=w667) -> (x .or. y?=w669:bool)
        n254 = case shown="True" w669 {
          tunnel: [w676 w682] -> w662
          tunnel: "Output Directory" -> [w676 w680]
          tunnel: [FALSE ("cancelled") w677] -> w664
          frame False {
          }
          frame True {
            n255 = Strip Path(path=w680) -> (stripped path=w679:path, name=w678:string)
            n256 = File Dialog(7:"Please Select a new or existing Results folder" ("prompt"), 9:w678, 11:w679) -> (1:w677:bool, 3:w682:path)  [unwired: 1 in, 5 out]
          }
        }
        n257 = local write "Output Directory"(w662) -> ()
        n258 = Not(x=w664) -> (.not. x?=w663:bool)
      }
      frame "Save Phase locked data" {
        n259 = global read "Meas_global.vi" "Raw data file"() -> (w687:path)
        n260 = stacked-sequence {
          seq-local: [_ w730 _ _] -> [_ _ _ w787]
          seq-local: [w704 _ _ _] -> [_ _ _ w788]
          seq-local: [_ _ w746 _] -> [_ _ _ w786]
          seq-local: [w693 _ _ _] -> [_ _ w744 _]
          tunnel: w689 -> [_ _ _ _]
          tunnel: w687 -> [w703 _ _ w792]
          tunnel: w685 -> [w700 _ _ _]
          tunnel: w684 -> [w699 _ _ _]
          tunnel: w683 -> [_ _ w743 _]
          frame #0 {
            w705 = "\r"
            n261 = local read "Number of Revs"() -> (w698:i32)
            n262 = Array Subset(array=w699, index (row)=1 ("index")) -> (w696:dbl[][])  [unwired: 3 in]
            n263 = Array Subset(array=w700, index (row)=1 ("index")) -> (w697:dbl[][])  [unwired: 3 in]
            n264 = for {
              tunnel: w698 -> [w713]
              tunnel: w697 -> [w712] mode=indexing
              tunnel: w696 -> [w711] mode=indexing
              tunnel: [w709] -> w695 mode=indexing
              tunnel: [w708] -> w694 mode=indexing
              n265 = Divide(x=w712, y=w713) -> (x/y=w709:dbl[])
              n266 = Divide(x=w711, y=w713) -> (x/y=w710:dbl[])
              n267 = Multiply(x=w709, y=w709) -> (x*y=w714:dbl[])
              n268 = Subtract(x=w710, y=w714) -> (x-y=w708:dbl[])
            }
            n269 = call "Read_RD_Ch_header.vi"("Raw data file"=w703) -> ("Ch string"=w707:string)  [unwired: 3 out]
            n270 = Build Array (concatenate)(w695, w694) -> (w693:dbl[][])
            n271 = Concatenate Strings(w705, "*****This is a many rows per single point file*****", w705, w707) -> (w704:string)
          }
          frame #1 {
            w716 = "\r"
            n272 = local read "Channel to Phase lock"() -> (w732:i32[])
            n273 = property on="Channel to Phase lock" class="LstBox (strict)"() -> ("Item Names"=w731:string[])  [unwired: 2 in, 2 out]
            n274 = Initialize Array("", 10) -> (w733:string[])
            n275 = call "Asterisk_header.vi"("Channel names"=w733) -> ("Header string"=w715:string)
            n276 = for {
              tunnel: w732 -> [w741] mode=indexing
              tunnel: w731 -> [w740]
              tunnel: [w739] -> w728 mode=indexing
              tunnel: ["Mean" ("format string")] -> w726 mode=indexing
              tunnel: ["Variance" ("format string")] -> w725 mode=indexing
              tunnel: [""] -> w723 mode=indexing
              n277 = Index Array(array=w740, index=w741) -> (element=w739:string)
            }
            n278 = Build Array (concatenate)("Rotor", w728, w728) -> (w722:string[])
            n279 = Build Array (concatenate)("Angle", w726, w725) -> (w721:string[])
            n280 = Build Array (concatenate)("(deg)", w723, w723) -> (w720:string[])
            n281 = Build Array(w722, w721, w720) -> (w719:string[][])
            n282 = Array To Spreadsheet String(array=w719, 3:"%s" ("format string")) -> (spreadsheet string=w717:string)  [unwired: 1 out]
            n283 = Concatenate Strings(w716, w715, w717, w716) -> (w730:string)
          }
          frame #2 {
            n284 = Array Size(array=w744) -> (size(s)=w747:i32[])
            n285 = Index Array(array=w747, index=0) -> (element=w753:i32)
            n286 = Divide(x=360, y=w743) -> (x/y=w742:dbl)
            n287 = Index Array(array=w747, index=1) -> (element=w748:i32)
            n288 = Decrement(x=w753) -> (x-1=w754:i32)
            n289 = for {
              N: w748 -> [_]
              shift-right: [w767] -> w746
              shift-left: "" -> [w762]
              tunnel: "Separation Character" -> [w758]
              tunnel: w744 -> [w765]
              tunnel: w754 -> [w761]
              tunnel: w742 -> [w760]
              i -> [w757]
              n290 = Index Array(array=w765, index (col)=w757) -> (element=w764:dbl[])  [unwired: 1 in]
              n291 = Multiply(x=w757, y=w760) -> (x*y=w756:dbl)
              n292 = call "Number_2_string.vi"("number"=w756) -> ("String"=w755:string)  [unwired: 1 in]
              n293 = Concatenate Strings(w755, w758) -> (w759:string)
              n294 = for {
                shift-right: [w775] -> w763
                shift-left: w759 -> [w776]
                tunnel: w758 -> [w774]
                tunnel: w764 -> [w770] mode=indexing
                tunnel: w761 -> [w772]
                i -> [w773]
                n295 = Equal?(x=w773, y=w772) -> (x = y?=w771:bool)
                n296 = call "Number_2_string.vi"("precision"="precision", "number"=w770) -> ("String"=w769:string)
                n297 = case shown="True" w771 {
                  tunnel: w776 -> [w780 w783]
                  tunnel: w769 -> [w779 w782]
                  tunnel: [w778 w781] -> w775
                  tunnel: w774 -> [w777 _]
                  frame False {
                    n298 = Concatenate Strings(w780, w779, w777) -> (w778:string)
                  }
                  frame True {
                    n299 = Concatenate Strings(w783, w782) -> (w781:string)
                  }
                }
              }
              n300 = Concatenate Strings(w762, w763, "\r") -> (w767:string)
            }
          }
          frame #3 {
            w784 = FALSE  # append to file? (new file:F)
            n301 = Strip Path(path=w792) -> (name=w790:string)  [unwired: 1 out]
            n302 = local read "Output Directory"() -> (w791:path)
            n303 = Build Path(base path=w791, name or relative path=w790) -> (appended path=w789:path)
            n304 = Concatenate Strings(w788, w787, w786) -> (w785:string)
            n305 = call "Write_File_Simple.vi"("append to file? (new file:F)"=w784, "character string"=w785, "file path"=w789) -> ()  [unwired: 2 out]
          }
        }
      }
    }
  }
